vi "HEWH Elapsed Timer Grouping.vi"(6 "Timer D":dbl, 7 "Total Elapsed Time":dbl, 8 "error in (no error)":errorcluster, 9 "Timer C":dbl, 10 "Timer B":dbl, 11 "Timer A":dbl) -> (0 "error out":errorcluster, 3 "Timer":T1)   [LabVIEW 2023]
uses:
  Type Definitions/HEWH Timer.ctl
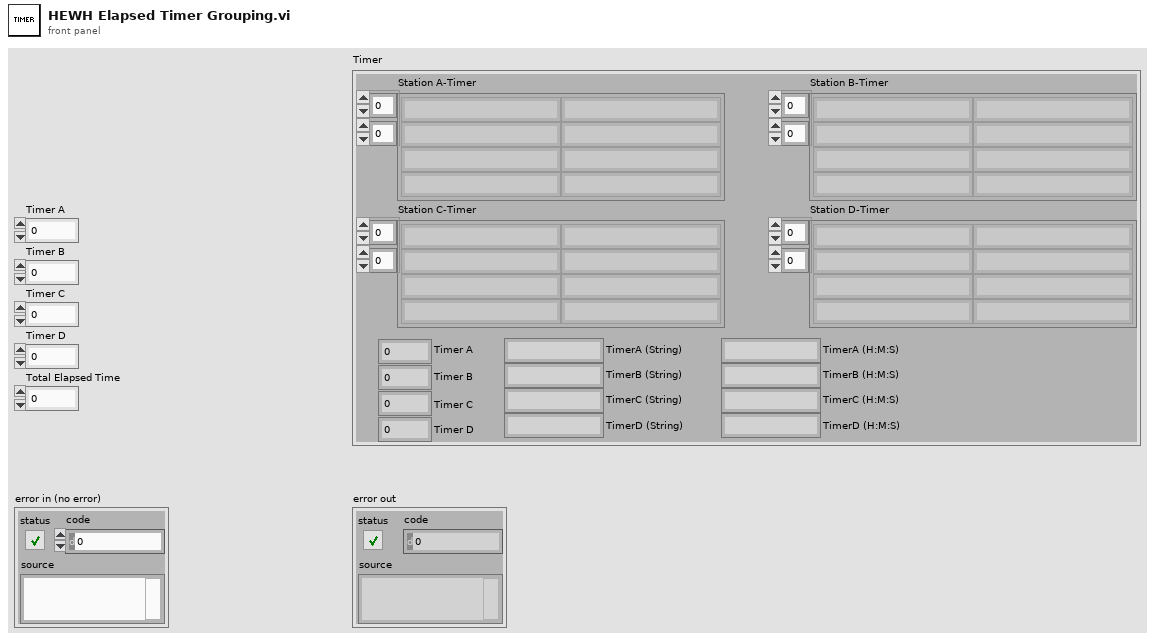
[diagram p1: front panel]
types:
  T1 = typedef "HEWH Timer.ctl" = cluster{"Station A-Timer":string[][], "Station B-Timer":string[][], "Station C-Timer":string[][], "Station D-Timer":string[][], "Timer A":dbl, "Timer B":dbl, "Timer C":dbl, "Timer D":dbl, "TimerA (String)":string, "TimerB (String)":string, "TimerC (String)":string, "TimerD (String)":string, "TimerA (H:M:S)":string, "TimerB (H:M:S)":string, "TimerC (H:M:S)":string, "TimerD (H:M:S)":string}
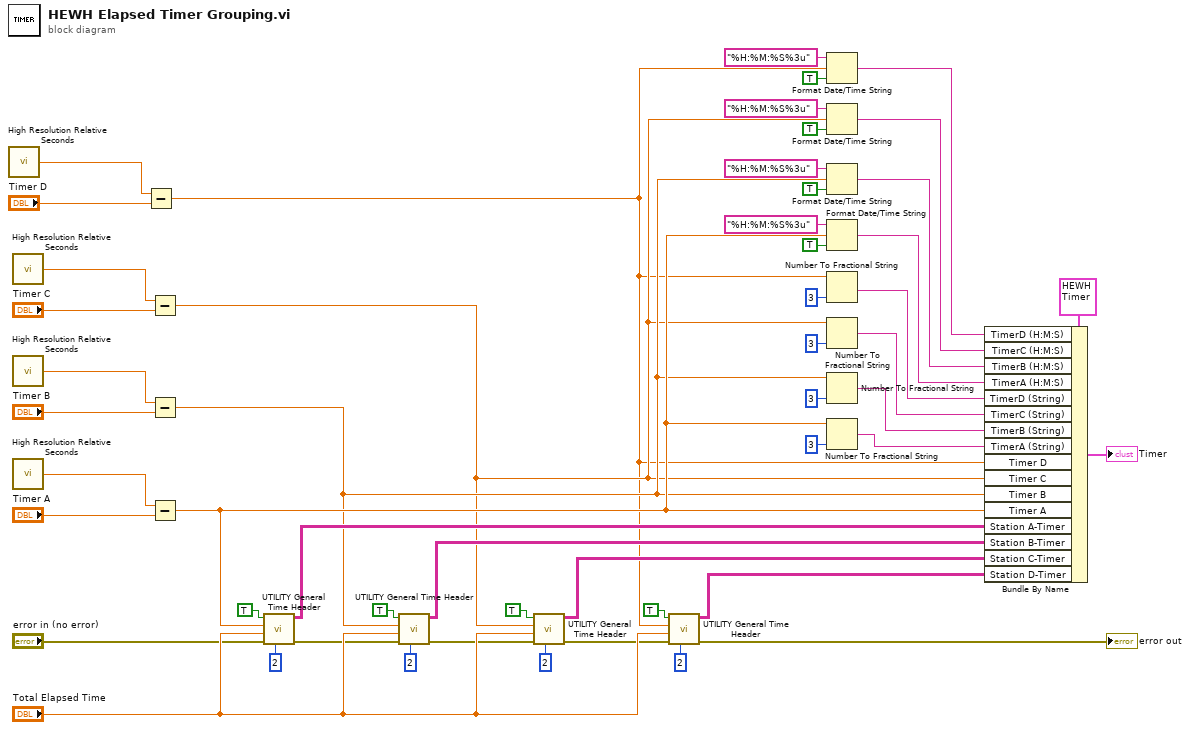
[diagram p0: block diagram]
diagram:
  n1 = call <vilib>:"High Resolution Relative Seconds.vi"() -> ("relative seconds"=w37:dbl)
  n2 = call <vilib>:"High Resolution Relative Seconds.vi"() -> ("relative seconds"=w35:dbl)
  n3 = call <vilib>:"High Resolution Relative Seconds.vi"() -> ("relative seconds"=w33:dbl)
  n4 = call <vilib>:"High Resolution Relative Seconds.vi"() -> ("relative seconds"=w31:dbl)
  n5 = Subtract(x=w37, y="Timer D") -> (x-y=w5:dbl)
  n6 = Subtract(x=w35, y="Timer C") -> (x-y=w6:dbl)
  n7 = Subtract(x=w33, y="Timer B") -> (x-y=w7:dbl)
  n8 = Subtract(x=w31, y="Timer A") -> (x-y=w8:dbl)
  n9 = call "UTILITY General Time Header.vi"("precision (6)"=i16 2, "Error In"="error in (no error)", "Software Elapsed Time"="Total Elapsed Time", "Elapsed Time"=w8, "Add Software Elapsed Time"=TRUE) -> ("Error Out"=w48:errorcluster, "Total Array"=w28:string[][])  [unwired: 5 in]
  n10 = call "UTILITY General Time Header.vi"("precision (6)"=i16 2, "Error In"=w48, "Software Elapsed Time"="Total Elapsed Time", "Elapsed Time"=w7, "Add Software Elapsed Time"=TRUE) -> ("Error Out"=w49:errorcluster, "Total Array"=w27:string[][])  [unwired: 5 in]
  n11 = call "UTILITY General Time Header.vi"("precision (6)"=i16 2, "Error In"=w49, "Software Elapsed Time"="Total Elapsed Time", "Elapsed Time"=w6, "Add Software Elapsed Time"=TRUE) -> ("Error Out"=w50:errorcluster, "Total Array"=w26:string[][])  [unwired: 5 in]
  n12 = call "UTILITY General Time Header.vi"("precision (6)"=i16 2, "Error In"=w50, "Software Elapsed Time"="Total Elapsed Time", "Elapsed Time"=w5, "Add Software Elapsed Time"=TRUE) -> ("Error Out"=→"error out":errorcluster, "Total Array"=w25:string[][])  [unwired: 5 in]
  n13 = Format Date/Time String(time format string (%c)="%H:%M:%S%3u", seconds (now)=w5, UTC format=TRUE) -> (date/time string=w4:string)
  n14 = Format Date/Time String(time format string (%c)="%H:%M:%S%3u", seconds (now)=w6, UTC format=TRUE) -> (date/time string=w3:string)
  n15 = Format Date/Time String(time format string (%c)="%H:%M:%S%3u", seconds (now)=w7, UTC format=TRUE) -> (date/time string=w2:string)
  n16 = Format Date/Time String(time format string (%c)="%H:%M:%S%3u", seconds (now)=w8, UTC format=TRUE) -> (date/time string=w1:string)
  n17 = Number To Fractional String(number=w5, precision (6)=i16 3) -> (F-format string=w15:string)  [unwired: 2 in]
  n18 = Number To Fractional String(number=w6, precision (6)=i16 3) -> (F-format string=w16:string)  [unwired: 2 in]
  n19 = Number To Fractional String(number=w7, precision (6)=i16 3) -> (F-format string=w17:string)  [unwired: 2 in]
  n20 = Number To Fractional String(number=w8, precision (6)=i16 3) -> (F-format string=w18:string)  [unwired: 2 in]
  n21 = Bundle By Name(cluster=T1 {"Station A-Timer"=[], "Station B-Timer"=[], "Station C-Timer"=[], "Station D-Timer"=[], "Timer A"=0.0, "Timer B"=0.0, "Timer C"=0.0, "Timer D"=0.0, "TimerA (String)"="", "TimerB (String)"="", "TimerC (String)"="", "TimerD (String)"="", "TimerA (H:M:S)"="", "TimerB (H:M:S)"="", "TimerC (H:M:S)"="", "TimerD (H:M:S)"=""} ("Timer"), "TimerD (H:M:S)"=w4, "TimerC (H:M:S)"=w3, "TimerB (H:M:S)"=w2, "TimerA (H:M:S)"=w1, "TimerD (String)"=w15, "TimerC (String)"=w16, "TimerB (String)"=w17, "TimerA (String)"=w18, "Timer D"=w5, "Timer C"=w6, "Timer B"=w7, "Timer A"=w8, "Station A-Timer"=w28, "Station B-Timer"=w27, "Station C-Timer"=w26, "Station D-Timer"=w25) -> (→"Timer":T1)
